vi "MaximumCut.vi"(0 "Tableau":dbl[][](array[numeric]) format="%.2f") -> (1 "Y Cut":dbl[](array[numeric]) format="%.2f", 2 "X Cut":dbl[](array[numeric]) format="%.2f")   [LabVIEW 2009]
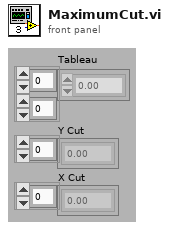
[diagram p1: front panel]
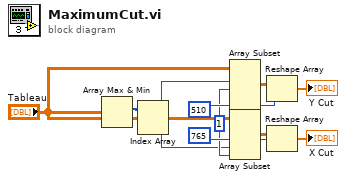
[diagram p0: block diagram]
diagram:
  w8 = 510
  w9 = 765
  w7 = 1
  n1 = Array Max & Min(array="Tableau") -> (max index (indices)=w6:i32[])  [unwired: 3 out]
  n2 = Index Array(array=w6) -> (element #1=w5:i32, element #2=w4:i32)  [unwired: 2 in]
  n3 = Array Subset(array="Tableau", index (row)=w5, length (row)=w7, length (col)=w8) -> (w11:dbl[][])  [unwired: 1 in]
  n4 = Array Subset(array="Tableau", length (row)=w9, index (col)=w4, length (col)=w7) -> (w10:dbl[][])  [unwired: 1 in]
  n5 = Reshape Array(w11, w8) -> (→"Y Cut":dbl[])
  n6 = Reshape Array(w10, w9) -> (→"X Cut":dbl[])
